vi "S4GUI_001.vi"() -> ()   [LabVIEW 2018] (continued)
                    n2026 = property on="Exptime ch3" class="DigNum (strict)"("Value"=w4669) -> ()  [unwired: 2 in, 2 out]
                  }
                }
                n2027 = call-dynamic "Read PREV_FT.vi"("error in (no error)"=w4601, "Interface in"=w4602) -> ("error out"=w4604:errorcluster, "PREV_FT"=w4603:bool, "Interface out"=w4605:refnum<class "Interface.lvclass">)  [unwired: 7 in]
                n2028 = call-dynamic "Get CCD_Config.vi"("error in (no error)"=w4604, "Interface in"=w4605) -> ("error out"=w4641:errorcluster, "output cluster"=w4640:T24, "Interface out"=w4644:refnum<class "Interface.lvclass">)  [unwired: 7 in]
                n2029 = Bundle By Name(cluster=w4640, "SHUTTER_MODE"=u8 1, "FRAME_TRANSFER"=w4603) -> (w4642:T24)
                n2030 = call-dynamic "Set CCD_Config.vi"("error in (no error)"=w4641, "input cluster"=w4642, "Interface in"=w4644) -> ("error out"=w4639:errorcluster, "Interface out"=w4645:refnum<class "Interface.lvclass">)  [unwired: 7 in]
                n2031 = Flatten To String(anything=w4642, error in (no error)=w4639) -> (data string=w4637:string, error out=w4638:errorcluster)  [unwired: 2 in, 1 out]
                n2032 = call "Write flatted cluster.vi"("error in (no error)"=w4638, "flatted cluster"=w4637, "Interface in"=w4645) -> ("error out"=w4647:errorcluster, "Interface out"=w4646:refnum<class "Interface.lvclass">)  [unwired: 7 in]
                n2033 = call-dynamic "Write Interface.vi"("error in (no error)"=w4647, "Interface.lvclass"=w4646, "Channel in"=w4633) -> ("error out"=w4652:errorcluster, "Channel out"=w4653:refnum<class "Channel.lvclass">)  [unwired: 7 in]
                n2034 = call "Write section_name.vi"("error in (no error)"=w4652, "section_name"="CCD_ACS3", "Channel in"=w4653) -> ("error out"=w4651:errorcluster, "Channel out"=w4656:refnum<class "Channel.lvclass">)  [unwired: 7 in]
                n2035 = call-dynamic "save config.vi"("error in (no error)"=w4651, "file config"="lastsaved.cfg", "Channel in"=w4656) -> ("error out"=w4610:errorcluster, "Channel out"=w4613:refnum<class "Channel.lvclass">)  [unwired: 7 in]
                n2036 = local read "Filter3"() -> (w4609:u8)
                n2037 = call-dynamic "Write Filter.vi"("error in (no error)"=w4610, "Filter"=w4609, "Channel in"=w4613) -> ("error out"=w4614:errorcluster, "Channel out"=w4627:refnum<class "Channel.lvclass">)  [unwired: 7 in]
                n2038 = call-dynamic "Read Interface.vi"("error in (no error)"=w4614, "Channel in"=w4627) -> ("error out"=w4617:errorcluster, "Interface.lvclass"=w4618:refnum<class "Interface.lvclass">, "Channel out"=w4628:refnum<class "Channel.lvclass">)  [unwired: 7 in]
                n2039 = call-dynamic "Write Suffix.vi"("error in (no error)"=w4617, "Suffix"=w4600, "Interface in"=w4618) -> ("error out"=w4626:errorcluster, "Interface out"=w4623:refnum<class "Interface.lvclass">)  [unwired: 7 in]
                n2040 = call-dynamic "Write ObsType.vi"("error in (no error)"=w4626, "ObsType"=w4599, "Interface in"=w4623) -> ("error out"=w4625:errorcluster, "Interface out"=w4622:refnum<class "Interface.lvclass">)  [unwired: 7 in]
                n2041 = call-dynamic "Write Object.vi"("error in (no error)"=w4625, "Object"=w4608, "Interface in"=w4622) -> ("error out"=w4624:errorcluster, "Interface out"=w4621:refnum<class "Interface.lvclass">)  [unwired: 7 in]
                n2042 = call-dynamic "Write Comments.vi"("error in (no error)"=w4624, "Comments"=w4607, "Interface in"=w4621) -> ("error out"=w4620:errorcluster, "Interface out"=w4619:refnum<class "Interface.lvclass">)  [unwired: 7 in]
                n2043 = call-dynamic "Write Observer.vi"("error in (no error)"=w4620, "Observer"=w4606, "Interface in"=w4619) -> ("error out"=w4615:errorcluster, "Interface out"=w4616:refnum<class "Interface.lvclass">)  [unwired: 7 in]
                n2044 = call-dynamic "Write Interface.vi"("error in (no error)"=w4615, "Interface.lvclass"=w4616, "Channel in"=w4628) -> ("error out"=w4611:errorcluster, "Channel out"=w4612:refnum<class "Channel.lvclass">)  [unwired: 7 in]
                n2045 = call-dynamic "Read State Machine.vi"("error in (no error)"=w4611, "Device in"=w4612) -> ("error out"=w4648:errorcluster, "State Machine.lvclass"=w4658:refnum<class "State Machine.lvclass">, "Device out"=w4657:refnum<class "Channel.lvclass">)  [unwired: 7 in]
                n2046 = call-dynamic "Write State.vi"("error in (no error)"=w4648, "State"=60, "State Machine in"=w4658) -> ("error out"=w4649:errorcluster, "State Machine out"=w4659:refnum<class "State Machine.lvclass">)  [unwired: 7 in]
                n2047 = call-dynamic "Write State Machine.vi"("error in (no error)"=w4649, "State Machine.lvclass"=w4659, "Device in"=w4657) -> ("error out"=w4661:errorcluster, "Device out"=w4660:refnum<class "Channel.lvclass">)  [unwired: 7 in]
                n2048 = call-dynamic "Write Channel.vi"("error in (no error)"=w4661, "Channel.lvclass"=w4660, "Acquisition in"=w4634) -> ("error out"=w4629:errorcluster, "Acquisition out"=w4630:refnum<class "Acquisition.lvclass">)  [unwired: 7 in]
              }
            }
          }
        }
        n2049 = call-dynamic "Write AcquisitionA.vi"("error in (no error)"=w3774, "Acquisition.lvclass"=w3775, "S4ACS_GUI in"=w3776) -> ("error out"=w3764:errorcluster, "S4ACS_GUI out"=w3768:refnum<class "S4GUI.lvclass">)  [unwired: 7 in]
        n2050 = call "Write AcquisitionB.vi"("error in (no error)"=w3769, "Acquisition.lvclass"=w3770, "S4ACS_GUI in"=w3768) -> ("error out"=w3763:errorcluster, "S4ACS_GUI out"=w3767:refnum<class "S4GUI.lvclass">)  [unwired: 7 in]
        n2051 = call-dynamic "Write AcquisitionC.vi"("error in (no error)"=w3758, "Acquisition.lvclass"=w3759, "S4ACS_GUI in"=w3767) -> ("error out"=w3762:errorcluster, "S4ACS_GUI out"=w3766:refnum<class "S4GUI.lvclass">)  [unwired: 7 in]
        n2052 = call-dynamic "Write AcquisitionD.vi"("error in (no error)"=w3756, "Acquisition.lvclass"=w3757, "S4ACS_GUI in"=w3766) -> ("error out"=w3761:errorcluster, "S4ACS_GUI out"=w3765:refnum<class "S4GUI.lvclass">)  [unwired: 7 in]
        n2053 = Merge Errors(w3764, w3763, w3762, w3761) -> (w3760:errorcluster)
        n2054 = call "Write cfg file.vi"("error in (no error)"=w3760, "cfg file"="lastsaved.cfg", "S4ACS_GUI in"=w3765) -> ("error out"=w3772:errorcluster, "S4ACS_GUI out"=w3771:refnum<class "S4GUI.lvclass">)  [unwired: 7 in]
      }
      event "set keywords": Value Change {
        # "SET Observer, suffix, comments e object da aba selecionada."
        n2055 = event-data() -> ()  [unwired: 1 in, 1 out]
        n2056 = local read "Tab Acq Type"() -> (w4846:T1)
        n2057 = local read "Observer"() -> (w4848:string)
        n2058 = case shown="\"ZERO\"" w4846 {
          tunnel: ["OBJECT" "FLAT" "FLAT" "DARK" "ZERO" "FOCUS"] -> w4852
          tunnel: [w5044 w5048 w5052 w5056 w5060 w5064] -> w4851
          tunnel: [w5043 w5047 w5051 w5055 w5059 w5063] -> w4850
          tunnel: [w5042 w5046 w5050 w5054 w5058 w5062] -> w4849
          frame "OBJECT", Default {
            n2059 = local read "Object_obj"() -> (w5044:string)
            n2060 = local read "OBJECT Comments"() -> (w5042:string)
            n2061 = local read "object suffix"() -> (w5043:string)
          }
          frame "DFLAT" {
            n2062 = local read "DFLAT Comments"() -> (w5046:string)
            n2063 = local read "Object_dflat"() -> (w5048:string)
            n2064 = local read "dflat suffix"() -> (w5047:string)
          }
          frame "SFLAT" {
            n2065 = local read "SFLAT Comments"() -> (w5050:string)
            n2066 = local read "Object_sflat"() -> (w5052:string)
            n2067 = local read "sflat suffix"() -> (w5051:string)
          }
          frame "DARK" {
            n2068 = local read "Object_dark"() -> (w5056:string)
            n2069 = local read "dark suffix"() -> (w5055:string)
            n2070 = local read "DARK Comments"() -> (w5054:string)
          }
          frame "ZERO" {
            n2071 = local read "ZERO Comments"() -> (w5058:string)
            n2072 = local read "Object_zero"() -> (w5060:string)
            n2073 = local read "zero suffix"() -> (w5059:string)
          }
          frame "FOCUS" {
            n2074 = local read "FOCUS Comments"() -> (w5062:string)
            n2075 = local read "Object_focus"() -> (w5064:string)
            n2076 = local read "focus suffix"() -> (w5063:string)
          }
        }
        n2077 = call-dynamic "Read AcquisitionC.vi"("error in (no error)"=w4832, "S4ACS_GUI in"=w4833) -> ("error out"=w4855:errorcluster, "Acquisition.lvclass"=w4856:refnum<class "Acquisition.lvclass">)  [unwired: 7 in, 1 out]
        n2078 = call-dynamic "Read AcquisitionA.vi"("error in (no error)"=w4832, "S4ACS_GUI in"=w4833) -> ("error out"=w4859:errorcluster, "Acquisition.lvclass"=w4860:refnum<class "Acquisition.lvclass">, "S4ACS_GUI out"=w4881:refnum<class "S4GUI.lvclass">)  [unwired: 7 in]
        n2079 = call "Read AcquisitionB.vi"("error in (no error)"=w4832, "S4ACS_GUI in"=w4833) -> ("error out"=w4857:errorcluster, "Acquisition.lvclass"=w4858:refnum<class "Acquisition.lvclass">)  [unwired: 7 in, 1 out]
        n2080 = call-dynamic "Read AcquisitionD.vi"("error in (no error)"=w4832, "S4ACS_GUI in"=w4833) -> ("error out"=w4853:errorcluster, "Acquisition.lvclass"=w4854:refnum<class "Acquisition.lvclass">)  [unwired: 7 in, 1 out]
        n2081 = call "Read connection.vi"("error in (no error)"=w4853, "Server in"=w4854) -> ("error out"=w4835:errorcluster, "connection"=w4834:bool, "Server out"=w4836:refnum<class "Acquisition.lvclass">)  [unwired: 7 in]
        n2082 = call "Read connection.vi"("error in (no error)"=w4855, "Server in"=w4856) -> ("error out"=w4838:errorcluster, "connection"=w4837:bool, "Server out"=w4839:refnum<class "Acquisition.lvclass">)  [unwired: 7 in]
        n2083 = call "Read connection.vi"("error in (no error)"=w4857, "Server in"=w4858) -> ("error out"=w4841:errorcluster, "connection"=w4840:bool, "Server out"=w4842:refnum<class "Acquisition.lvclass">)  [unwired: 7 in]
        n2084 = call "Read connection.vi"("error in (no error)"=w4859, "Server in"=w4860) -> ("error out"=w4844:errorcluster, "connection"=w4843:bool, "Server out"=w4845:refnum<class "Acquisition.lvclass">)  [unwired: 7 in]
        n2085 = To Lower Case(string=w4850) -> (all lower case string=w4847:string)
        n2086 = case shown="True" w4840 {
          tunnel: w4842 -> [w4963 w4992]
          tunnel: w4841 -> [w4962 w4991]
          tunnel: [w4963 w4990] -> w4875
          tunnel: [w4962 w4989] -> w4874
          tunnel: w4847 -> [_ w4970]
          tunnel: w4852 -> [_ w4969]
          tunnel: w4851 -> [_ w4968]
          tunnel: w4849 -> [_ w4967]
          tunnel: w4848 -> [_ w4966]
          frame False {
          }
          frame True {
            n2087 = call-dynamic "Read Channel.vi"("error in (no error)"=w4991, "Acquisition in"=w4992) -> ("error out"=w4964:errorcluster, "Channel.lvclass"=w4965:refnum<class "Channel.lvclass">, "Acquisition out"=w4993:refnum<class "Acquisition.lvclass">)  [unwired: 7 in]
            n2088 = local read "Filter2"() -> (w4971:u8)
            n2089 = call-dynamic "Write Filter.vi"("error in (no error)"=w4964, "Filter"=w4971, "Channel in"=w4965) -> ("error out"=w4988:errorcluster, "Channel out"=w4975:refnum<class "Channel.lvclass">)  [unwired: 7 in]
            n2090 = call-dynamic "Read Interface.vi"("error in (no error)"=w4988, "Channel in"=w4975) -> ("error out"=w4985:errorcluster, "Interface.lvclass"=w4984:refnum<class "Interface.lvclass">, "Channel out"=w4974:refnum<class "Channel.lvclass">)  [unwired: 7 in]
            n2091 = call-dynamic "Write Suffix.vi"("error in (no error)"=w4985, "Suffix"=w4970, "Interface in"=w4984) -> ("error out"=w4976:errorcluster, "Interface out"=w4979:refnum<class "Interface.lvclass">)  [unwired: 7 in]
            n2092 = call-dynamic "Write ObsType.vi"("error in (no error)"=w4976, "ObsType"=w4969, "Interface in"=w4979) -> ("error out"=w4977:errorcluster, "Interface out"=w4980:refnum<class "Interface.lvclass">)  [unwired: 7 in]
            n2093 = call-dynamic "Write Object.vi"("error in (no error)"=w4977, "Object"=w4968, "Interface in"=w4980) -> ("error out"=w4978:errorcluster, "Interface out"=w4981:refnum<class "Interface.lvclass">)  [unwired: 7 in]
            n2094 = call-dynamic "Write Comments.vi"("error in (no error)"=w4978, "Comments"=w4967, "Interface in"=w4981) -> ("error out"=w4982:errorcluster, "Interface out"=w4983:refnum<class "Interface.lvclass">)  [unwired: 7 in]
            n2095 = call-dynamic "Write Observer.vi"("error in (no error)"=w4982, "Observer"=w4966, "Interface in"=w4983) -> ("error out"=w4987:errorcluster, "Interface out"=w4986:refnum<class "Interface.lvclass">)  [unwired: 7 in]
            n2096 = call-dynamic "Write Interface.vi"("error in (no error)"=w4987, "Interface.lvclass"=w4986, "Channel in"=w4974) -> ("error out"=w4972:errorcluster, "Channel out"=w4973:refnum<class "Channel.lvclass">)  [unwired: 7 in]
            n2097 = call-dynamic "Read State Machine.vi"("error in (no error)"=w4972, "Device in"=w4973) -> ("error out"=w4994:errorcluster, "State Machine.lvclass"=w4998:refnum<class "State Machine.lvclass">, "Device out"=w4997:refnum<class "Channel.lvclass">)  [unwired: 7 in]
            n2098 = call-dynamic "Write State.vi"("error in (no error)"=w4994, "State"=12, "State Machine in"=w4998) -> ("error out"=w4995:errorcluster, "State Machine out"=w4999:refnum<class "State Machine.lvclass">)  [unwired: 7 in]
            n2099 = call-dynamic "Write State Machine.vi"("error in (no error)"=w4995, "State Machine.lvclass"=w4999, "Device in"=w4997) -> ("error out"=w5001:errorcluster, "Device out"=w5000:refnum<class "Channel.lvclass">)  [unwired: 7 in]
            n2100 = call-dynamic "Write Channel.vi"("error in (no error)"=w5001, "Channel.lvclass"=w5000, "Acquisition in"=w4993) -> ("error out"=w4989:errorcluster, "Acquisition out"=w4990:refnum<class "Acquisition.lvclass">)  [unwired: 7 in]
          }
        }
        n2101 = case shown="True" w4843 {
          tunnel: [w5002 w5040] -> w4879
          tunnel: [w5003 w5039] -> w4880
          tunnel: w4845 -> [w5003 w5030]
          tunnel: w4844 -> [w5002 w5029]
          tunnel: w4847 -> [_ w5010]
          tunnel: w4852 -> [_ w5009]
          tunnel: w4851 -> [_ w5008]
          tunnel: w4849 -> [_ w5007]
          tunnel: w4848 -> [_ w5006]
          frame False {
          }
          frame True {
            n2102 = call-dynamic "Read Channel.vi"("error in (no error)"=w5029, "Acquisition in"=w5030) -> ("error out"=w5004:errorcluster, "Channel.lvclass"=w5005:refnum<class "Channel.lvclass">, "Acquisition out"=w5041:refnum<class "Acquisition.lvclass">)  [unwired: 7 in]
            n2103 = local read "Filter1"() -> (w5013:u8)
            n2104 = call-dynamic "Write Filter.vi"("error in (no error)"=w5004, "Filter"=w5013, "Channel in"=w5005) -> ("error out"=w5028:errorcluster, "Channel out"=w5027:refnum<class "Channel.lvclass">)  [unwired: 7 in]
            n2105 = call-dynamic "Read Interface.vi"("error in (no error)"=w5028, "Channel in"=w5027) -> ("error out"=w5024:errorcluster, "Interface.lvclass"=w5023:refnum<class "Interface.lvclass">, "Channel out"=w5017:refnum<class "Channel.lvclass">)  [unwired: 7 in]
            n2106 = call-dynamic "Write Suffix.vi"("error in (no error)"=w5024, "Suffix"=w5010, "Interface in"=w5023) -> ("error out"=w5014:errorcluster, "Interface out"=w5018:refnum<class "Interface.lvclass">)  [unwired: 7 in]
            n2107 = call-dynamic "Write ObsType.vi"("error in (no error)"=w5014, "ObsType"=w5009, "Interface in"=w5018) -> ("error out"=w5015:errorcluster, "Interface out"=w5019:refnum<class "Interface.lvclass">)  [unwired: 7 in]
            n2108 = call-dynamic "Write Object.vi"("error in (no error)"=w5015, "Object"=w5008, "Interface in"=w5019) -> ("error out"=w5016:errorcluster, "Interface out"=w5020:refnum<class "Interface.lvclass">)  [unwired: 7 in]
            n2109 = call-dynamic "Write Comments.vi"("error in (no error)"=w5016, "Comments"=w5007, "Interface in"=w5020) -> ("error out"=w5021:errorcluster, "Interface out"=w5022:refnum<class "Interface.lvclass">)  [unwired: 7 in]
            n2110 = call-dynamic "Write Observer.vi"("error in (no error)"=w5021, "Observer"=w5006, "Interface in"=w5022) -> ("error out"=w5026:errorcluster, "Interface out"=w5025:refnum<class "Interface.lvclass">)  [unwired: 7 in]
            n2111 = call-dynamic "Write Interface.vi"("error in (no error)"=w5026, "Interface.lvclass"=w5025, "Channel in"=w5017) -> ("error out"=w5011:errorcluster, "Channel out"=w5012:refnum<class "Channel.lvclass">)  [unwired: 7 in]
            n2112 = call-dynamic "Read State Machine.vi"("error in (no error)"=w5011, "Device in"=w5012) -> ("error out"=w5038:errorcluster, "State Machine.lvclass"=w5034:refnum<class "State Machine.lvclass">, "Device out"=w5035:refnum<class "Channel.lvclass">)  [unwired: 7 in]
            n2113 = call-dynamic "Write State.vi"("error in (no error)"=w5038, "State"=12, "State Machine in"=w5034) -> ("error out"=w5037:errorcluster, "State Machine out"=w5033:refnum<class "State Machine.lvclass">)  [unwired: 7 in]
            n2114 = call-dynamic "Write State Machine.vi"("error in (no error)"=w5037, "State Machine.lvclass"=w5033, "Device in"=w5035) -> ("error out"=w5031:errorcluster, "Device out"=w5032:refnum<class "Channel.lvclass">)  [unwired: 7 in]
            n2115 = call-dynamic "Write Channel.vi"("error in (no error)"=w5031, "Channel.lvclass"=w5032, "Acquisition in"=w5041) -> ("error out"=w5040:errorcluster, "Acquisition out"=w5039:refnum<class "Acquisition.lvclass">)  [unwired: 7 in]
          }
        }
        n2116 = case shown="True" w4837 {
          tunnel: w4839 -> [w4923 w4952]
          tunnel: w4838 -> [w4922 w4951]
          tunnel: [w4923 w4950] -> w4864
          tunnel: [w4922 w4949] -> w4863
          tunnel: w4847 -> [_ w4930]
          tunnel: w4852 -> [_ w4929]
          tunnel: w4851 -> [_ w4928]
          tunnel: w4849 -> [_ w4927]
          tunnel: w4848 -> [_ w4926]
          frame False {
          }
          frame True {
            n2117 = call-dynamic "Read Channel.vi"("error in (no error)"=w4951, "Acquisition in"=w4952) -> ("error out"=w4924:errorcluster, "Channel.lvclass"=w4925:refnum<class "Channel.lvclass">, "Acquisition out"=w4953:refnum<class "Acquisition.lvclass">)  [unwired: 7 in]
            n2118 = local read "Filter3"() -> (w4931:u8)
            n2119 = call-dynamic "Write Filter.vi"("error in (no error)"=w4924, "Filter"=w4931, "Channel in"=w4925) -> ("error out"=w4934:errorcluster, "Channel out"=w4947:refnum<class "Channel.lvclass">)  [unwired: 7 in]
            n2120 = call-dynamic "Read Interface.vi"("error in (no error)"=w4934, "Channel in"=w4947) -> ("error out"=w4937:errorcluster, "Interface.lvclass"=w4938:refnum<class "Interface.lvclass">, "Channel out"=w4948:refnum<class "Channel.lvclass">)  [unwired: 7 in]
            n2121 = call-dynamic "Write Suffix.vi"("error in (no error)"=w4937, "Suffix"=w4930, "Interface in"=w4938) -> ("error out"=w4946:errorcluster, "Interface out"=w4943:refnum<class "Interface.lvclass">)  [unwired: 7 in]
            n2122 = call-dynamic "Write ObsType.vi"("error in (no error)"=w4946, "ObsType"=w4929, "Interface in"=w4943) -> ("error out"=w4945:errorcluster, "Interface out"=w4942:refnum<class "Interface.lvclass">)  [unwired: 7 in]
            n2123 = call-dynamic "Write Object.vi"("error in (no error)"=w4945, "Object"=w4928, "Interface in"=w4942) -> ("error out"=w4944:errorcluster, "Interface out"=w4941:refnum<class "Interface.lvclass">)  [unwired: 7 in]
            n2124 = call-dynamic "Write Comments.vi"("error in (no error)"=w4944, "Comments"=w4927, "Interface in"=w4941) -> ("error out"=w4940:errorcluster, "Interface out"=w4939:refnum<class "Interface.lvclass">)  [unwired: 7 in]
            n2125 = call-dynamic "Write Observer.vi"("error in (no error)"=w4940, "Observer"=w4926, "Interface in"=w4939) -> ("error out"=w4935:errorcluster, "Interface out"=w4936:refnum<class "Interface.lvclass">)  [unwired: 7 in]
            n2126 = call-dynamic "Write Interface.vi"("error in (no error)"=w4935, "Interface.lvclass"=w4936, "Channel in"=w4948) -> ("error out"=w4932:errorcluster, "Channel out"=w4933:refnum<class "Channel.lvclass">)  [unwired: 7 in]
            n2127 = call-dynamic "Read State Machine.vi"("error in (no error)"=w4932, "Device in"=w4933) -> ("error out"=w4954:errorcluster, "State Machine.lvclass"=w4958:refnum<class "State Machine.lvclass">, "Device out"=w4957:refnum<class "Channel.lvclass">)  [unwired: 7 in]
            n2128 = call-dynamic "Write State.vi"("error in (no error)"=w4954, "State"=12, "State Machine in"=w4958) -> ("error out"=w4955:errorcluster, "State Machine out"=w4959:refnum<class "State Machine.lvclass">)  [unwired: 7 in]
            n2129 = call-dynamic "Write State Machine.vi"("error in (no error)"=w4955, "State Machine.lvclass"=w4959, "Device in"=w4957) -> ("error out"=w4961:errorcluster, "Device out"=w4960:refnum<class "Channel.lvclass">)  [unwired: 7 in]
            n2130 = call-dynamic "Write Channel.vi"("error in (no error)"=w4961, "Channel.lvclass"=w4960, "Acquisition in"=w4953) -> ("error out"=w4949:errorcluster, "Acquisition out"=w4950:refnum<class "Acquisition.lvclass">)  [unwired: 7 in]
          }
        }
        n2131 = case shown="True" w4834 {
          tunnel: w4836 -> [w4883 w4912]
          tunnel: w4835 -> [w4882 w4911]
          tunnel: [w4883 w4910] -> w4862
          tunnel: [w4882 w4909] -> w4861
          tunnel: w4847 -> [_ w4890]
          tunnel: w4852 -> [_ w4889]
          tunnel: w4851 -> [_ w4888]
          tunnel: w4849 -> [_ w4887]
          tunnel: w4848 -> [_ w4886]
          frame False {
          }
          frame True {
            n2132 = call-dynamic "Read Channel.vi"("error in (no error)"=w4911, "Acquisition in"=w4912) -> ("error out"=w4884:errorcluster, "Channel.lvclass"=w4885:refnum<class "Channel.lvclass">, "Acquisition out"=w4921:refnum<class "Acquisition.lvclass">)  [unwired: 7 in]
            n2133 = local read "Filter4"() -> (w4891:u8)
            n2134 = call-dynamic "Write Filter.vi"("error in (no error)"=w4884, "Filter"=w4891, "Channel in"=w4885) -> ("error out"=w4908:errorcluster, "Channel out"=w4895:refnum<class "Channel.lvclass">)  [unwired: 7 in]
            n2135 = call-dynamic "Read Interface.vi"("error in (no error)"=w4908, "Channel in"=w4895) -> ("error out"=w4905:errorcluster, "Interface.lvclass"=w4904:refnum<class "Interface.lvclass">, "Channel out"=w4894:refnum<class "Channel.lvclass">)  [unwired: 7 in]
            n2136 = call-dynamic "Write Suffix.vi"("error in (no error)"=w4905, "Suffix"=w4890, "Interface in"=w4904) -> ("error out"=w4896:errorcluster, "Interface out"=w4899:refnum<class "Interface.lvclass">)  [unwired: 7 in]
            n2137 = call-dynamic "Write ObsType.vi"("error in (no error)"=w4896, "ObsType"=w4889, "Interface in"=w4899) -> ("error out"=w4897:errorcluster, "Interface out"=w4900:refnum<class "Interface.lvclass">)  [unwired: 7 in]
            n2138 = call-dynamic "Write Object.vi"("error in (no error)"=w4897, "Object"=w4888, "Interface in"=w4900) -> ("error out"=w4898:errorcluster, "Interface out"=w4901:refnum<class "Interface.lvclass">)  [unwired: 7 in]
            n2139 = call-dynamic "Write Comments.vi"("error in (no error)"=w4898, "Comments"=w4887, "Interface in"=w4901) -> ("error out"=w4902:errorcluster, "Interface out"=w4903:refnum<class "Interface.lvclass">)  [unwired: 7 in]
            n2140 = call-dynamic "Write Observer.vi"("error in (no error)"=w4902, "Observer"=w4886, "Interface in"=w4903) -> ("error out"=w4907:errorcluster, "Interface out"=w4906:refnum<class "Interface.lvclass">)  [unwired: 7 in]
            n2141 = call-dynamic "Write Interface.vi"("error in (no error)"=w4907, "Interface.lvclass"=w4906, "Channel in"=w4894) -> ("error out"=w4892:errorcluster, "Channel out"=w4893:refnum<class "Channel.lvclass">)  [unwired: 7 in]
            n2142 = call-dynamic "Read State Machine.vi"("error in (no error)"=w4892, "Device in"=w4893) -> ("error out"=w4920:errorcluster, "State Machine.lvclass"=w4916:refnum<class "State Machine.lvclass">, "Device out"=w4917:refnum<class "Channel.lvclass">)  [unwired: 7 in]
            n2143 = call-dynamic "Write State.vi"("error in (no error)"=w4920, "State"=12, "State Machine in"=w4916) -> ("error out"=w4919:errorcluster, "State Machine out"=w4915:refnum<class "State Machine.lvclass">)  [unwired: 7 in]
            n2144 = call-dynamic "Write State Machine.vi"("error in (no error)"=w4919, "State Machine.lvclass"=w4915, "Device in"=w4917) -> ("error out"=w4913:errorcluster, "Device out"=w4914:refnum<class "Channel.lvclass">)  [unwired: 7 in]
            n2145 = call-dynamic "Write Channel.vi"("error in (no error)"=w4913, "Channel.lvclass"=w4914, "Acquisition in"=w4921) -> ("error out"=w4909:errorcluster, "Acquisition out"=w4910:refnum<class "Acquisition.lvclass">)  [unwired: 7 in]
          }
        }
        n2146 = call-dynamic "Write AcquisitionA.vi"("error in (no error)"=w4879, "Acquisition.lvclass"=w4880, "S4ACS_GUI in"=w4881) -> ("error out"=w4869:errorcluster, "S4ACS_GUI out"=w4873:refnum<class "S4GUI.lvclass">)  [unwired: 7 in]
        n2147 = call "Write AcquisitionB.vi"("error in (no error)"=w4874, "Acquisition.lvclass"=w4875, "S4ACS_GUI in"=w4873) -> ("error out"=w4868:errorcluster, "S4ACS_GUI out"=w4872:refnum<class "S4GUI.lvclass">)  [unwired: 7 in]
        n2148 = call-dynamic "Write AcquisitionC.vi"("error in (no error)"=w4863, "Acquisition.lvclass"=w4864, "S4ACS_GUI in"=w4872) -> ("error out"=w4867:errorcluster, "S4ACS_GUI out"=w4871:refnum<class "S4GUI.lvclass">)  [unwired: 7 in]
        n2149 = call-dynamic "Write AcquisitionD.vi"("error in (no error)"=w4861, "Acquisition.lvclass"=w4862, "S4ACS_GUI in"=w4871) -> ("error out"=w4866:errorcluster, "S4ACS_GUI out"=w4870:refnum<class "S4GUI.lvclass">)  [unwired: 7 in]
        n2150 = Merge Errors(w4869, w4868, w4867, w4866) -> (w4865:errorcluster)
        n2151 = call "Write cfg file.vi"("error in (no error)"=w4865, "cfg file"="lastsaved.cfg", "S4ACS_GUI in"=w4870) -> ("error out"=w4877:errorcluster, "S4ACS_GUI out"=w4876:refnum<class "S4GUI.lvclass">)  [unwired: 7 in]
      }
      event "Object_sflat", "Object_dark", "Object_zero", "Object_dflat", "Object_focus", "Object_obj": Value Change {
        n2152 = event-data() -> ("NewVal"=w5066:string)  [unwired: 1 in, 5 out]
        n2153 = stacked-sequence {
          seq-local: [w5102 _ _ _] -> [_ w5160 _ _]
          seq-local: [w5101 _ _ _] -> [_ w5159 _ _]
          seq-local: [_ w5158 _ _] -> [_ _ w5203 _]
          seq-local: [_ w5157 _ _] -> [_ _ w5202 _]
          seq-local: [_ _ w5201 _] -> [_ _ _ w5246]
          seq-local: [_ _ w5200 _] -> [_ _ _ w5245]
          tunnel: w5073 -> [w5114 _ _ _]
          tunnel: w5074 -> [w5113 _ _ _]
          tunnel: [_ _ _ w5244] -> w5068
          tunnel: [_ _ _ w5243] -> w5067
          tunnel: w5072 -> [w5100 w5156 w5199 w5242]
          tunnel: w5071 -> [w5099 w5155 w5185 w5228]
          tunnel: w5069 -> [w5098 w5141 w5184 w5227]
          tunnel: w5066 -> [w5097 w5140 w5183 w5226]
          tunnel: w5070 -> [w5096 w5139 w5182 w5225]
          frame #0 {
            # "observer"
            # "comment"
            # "object"
            # "suffix"
            # "obsType"
            n2154 = call-dynamic "Read AcquisitionA.vi"("error in (no error)"=w5114, "S4ACS_GUI in"=w5113) -> ("error out"=w5112:errorcluster, "Acquisition.lvclass"=w5111:refnum<class "Acquisition.lvclass">, "S4ACS_GUI out"=w5106:refnum<class "S4GUI.lvclass">)  [unwired: 7 in]
            n2155 = call-dynamic "Read Channel.vi"("error in (no error)"=w5112, "Acquisition in"=w5111) -> ("error out"=w5076:errorcluster, "Channel.lvclass"=w5079:refnum<class "Channel.lvclass">, "Acquisition out"=w5105:refnum<class "Acquisition.lvclass">)  [unwired: 7 in]
            n2156 = local read "Filter1"() -> (w5077:u8)
            n2157 = call-dynamic "Write Filter.vi"("error in (no error)"=w5076, "Filter"=w5077, "Channel in"=w5079) -> ("error out"=w5075:errorcluster, "Channel out"=w5078:refnum<class "Channel.lvclass">)  [unwired: 7 in]
            n2158 = call-dynamic "Read Interface.vi"("error in (no error)"=w5075, "Channel in"=w5078) -> ("error out"=w5092:errorcluster, "Interface.lvclass"=w5093:refnum<class "Interface.lvclass">, "Channel out"=w5110:refnum<class "Channel.lvclass">)  [unwired: 7 in]
            n2159 = call-dynamic "Write Suffix.vi"("error in (no error)"=w5092, "Suffix"=w5100, "Interface in"=w5093) -> ("error out"=w5117:errorcluster, "Interface out"=w5109:refnum<class "Interface.lvclass">)  [unwired: 7 in]
            n2160 = call-dynamic "Write ObsType.vi"("error in (no error)"=w5117, "ObsType"=w5098, "Interface in"=w5109) -> ("error out"=w5116:errorcluster, "Interface out"=w5108:refnum<class "Interface.lvclass">)  [unwired: 7 in]
            n2161 = call-dynamic "Write Object.vi"("error in (no error)"=w5116, "Object"=w5097, "Interface in"=w5108) -> ("error out"=w5115:errorcluster, "Interface out"=w5107:refnum<class "Interface.lvclass">)  [unwired: 7 in]
            n2162 = call-dynamic "Write Comments.vi"("error in (no error)"=w5115, "Comments"=w5099, "Interface in"=w5107) -> ("error out"=w5095:errorcluster, "Interface out"=w5094:refnum<class "Interface.lvclass">)  [unwired: 7 in]
            n2163 = call-dynamic "Write Observer.vi"("error in (no error)"=w5095, "Observer"=w5096, "Interface in"=w5094) -> ("error out"=w5090:errorcluster, "Interface out"=w5091:refnum<class "Interface.lvclass">)  [unwired: 7 in]
            n2164 = call-dynamic "Write Interface.vi"("error in (no error)"=w5090, "Interface.lvclass"=w5091, "Channel in"=w5110) -> ("error out"=w5086:errorcluster, "Channel out"=w5089:refnum<class "Channel.lvclass">)  [unwired: 7 in]
            n2165 = call-dynamic "Read State Machine.vi"("error in (no error)"=w5086, "Device in"=w5089) -> ("error out"=w5085:errorcluster, "State Machine.lvclass"=w5083:refnum<class "State Machine.lvclass">, "Device out"=w5088:refnum<class "Channel.lvclass">)  [unwired: 7 in]
            n2166 = call "Next State.vi"("error in (no error)"=w5085, "New_State"=12, "State Machine in"=w5083) -> ("error out"=w5084:errorcluster, "State Machine out"=w5082:refnum<class "State Machine.lvclass">)  [unwired: 7 in]
            n2167 = call-dynamic "Write State Machine.vi"("error in (no error)"=w5084, "State Machine.lvclass"=w5082, "Device in"=w5088) -> ("error out"=w5081:errorcluster, "Device out"=w5087:refnum<class "Channel.lvclass">)  [unwired: 7 in]
            n2168 = call-dynamic "Write Channel.vi"("error in (no error)"=w5081, "Channel.lvclass"=w5087, "Acquisition in"=w5105) -> ("error out"=w5103:errorcluster, "Acquisition out"=w5104:refnum<class "Acquisition.lvclass">)  [unwired: 7 in]
            n2169 = call-dynamic "Write AcquisitionA.vi"("error in (no error)"=w5103, "Acquisition.lvclass"=w5104, "S4ACS_GUI in"=w5106) -> ("error out"=w5101:errorcluster, "S4ACS_GUI out"=w5102:refnum<class "S4GUI.lvclass">)  [unwired: 7 in]
          }
          frame #1 {
            # "object"
            # "suffix"
            # "obsType"
            n2170 = call "Read AcquisitionB.vi"("error in (no error)"=w5159, "S4ACS_GUI in"=w5160) -> ("error out"=w5145:errorcluster, "Acquisition.lvclass"=w5146:refnum<class "Acquisition.lvclass">, "S4ACS_GUI out"=w5151:refnum<class "S4GUI.lvclass">)  [unwired: 7 in]
            n2171 = call-dynamic "Read Channel.vi"("error in (no error)"=w5145, "Acquisition in"=w5146) -> ("error out"=w5119:errorcluster, "Channel.lvclass"=w5121:refnum<class "Channel.lvclass">, "Acquisition out"=w5152:refnum<class "Acquisition.lvclass">)  [unwired: 7 in]
            n2172 = local read "Filter2"() -> (w5122:u8)
            n2173 = call-dynamic "Write Filter.vi"("error in (no error)"=w5119, "Filter"=w5122, "Channel in"=w5121) -> ("error out"=w5118:errorcluster, "Channel out"=w5120:refnum<class "Channel.lvclass">)  [unwired: 7 in]
            n2174 = call-dynamic "Read Interface.vi"("error in (no error)"=w5118, "Channel in"=w5120) -> ("error out"=w5133:errorcluster, "Interface.lvclass"=w5134:refnum<class "Interface.lvclass">, "Channel out"=w5147:refnum<class "Channel.lvclass">)  [unwired: 7 in]
            n2175 = call-dynamic "Write Suffix.vi"("error in (no error)"=w5133, "Suffix"=w5156, "Interface in"=w5134) -> ("error out"=w5142:errorcluster, "Interface out"=w5148:refnum<class "Interface.lvclass">)  [unwired: 7 in]
            n2176 = call-dynamic "Write ObsType.vi"("error in (no error)"=w5142, "ObsType"=w5141, "Interface in"=w5148) -> ("error out"=w5143:errorcluster, "Interface out"=w5149:refnum<class "Interface.lvclass">)  [unwired: 7 in]
            n2177 = call-dynamic "Write Object.vi"("error in (no error)"=w5143, "Object"=w5140, "Interface in"=w5149) -> ("error out"=w5144:errorcluster, "Interface out"=w5150:refnum<class "Interface.lvclass">)  [unwired: 7 in]
            n2178 = call-dynamic "Write Comments.vi"("error in (no error)"=w5144, "Comments"=w5155, "Interface in"=w5150) -> ("error out"=w5136:errorcluster, "Interface out"=w5135:refnum<class "Interface.lvclass">)  [unwired: 7 in]
            n2179 = call-dynamic "Write Observer.vi"("error in (no error)"=w5136, "Observer"=w5139, "Interface in"=w5135) -> ("error out"=w5137:errorcluster, "Interface out"=w5138:refnum<class "Interface.lvclass">)  [unwired: 7 in]
            n2180 = call-dynamic "Write Interface.vi"("error in (no error)"=w5137, "Interface.lvclass"=w5138, "Channel in"=w5147) -> ("error out"=w5126:errorcluster, "Channel out"=w5127:refnum<class "Channel.lvclass">)  [unwired: 7 in]
            n2181 = call-dynamic "Read State Machine.vi"("error in (no error)"=w5126, "Device in"=w5127) -> ("error out"=w5132:errorcluster, "State Machine.lvclass"=w5130:refnum<class "State Machine.lvclass">, "Device out"=w5125:refnum<class "Channel.lvclass">)  [unwired: 7 in]
            n2182 = call "Next State.vi"("error in (no error)"=w5132, "New_State"=12, "State Machine in"=w5130) -> ("error out"=w5131:errorcluster, "State Machine out"=w5129:refnum<class "State Machine.lvclass">)  [unwired: 7 in]
            n2183 = call-dynamic "Write State Machine.vi"("error in (no error)"=w5131, "State Machine.lvclass"=w5129, "Device in"=w5125) -> ("error out"=w5123:errorcluster, "Device out"=w5124:refnum<class "Channel.lvclass">)  [unwired: 7 in]
            n2184 = call-dynamic "Write Channel.vi"("error in (no error)"=w5123, "Channel.lvclass"=w5124, "Acquisition in"=w5152) -> ("error out"=w5154:errorcluster, "Acquisition out"=w5153:refnum<class "Acquisition.lvclass">)  [unwired: 7 in]
            n2185 = call "Write AcquisitionB.vi"("error in (no error)"=w5154, "Acquisition.lvclass"=w5153, "S4ACS_GUI in"=w5151) -> ("error out"=w5157:errorcluster, "S4ACS_GUI out"=w5158:refnum<class "S4GUI.lvclass">)  [unwired: 7 in]
          }
          frame #2 {
            # "object"
            # "suffix"
            # "obsType"
            n2186 = call-dynamic "Read AcquisitionC.vi"("error in (no error)"=w5202, "S4ACS_GUI in"=w5203) -> ("error out"=w5195:errorcluster, "Acquisition.lvclass"=w5194:refnum<class "Acquisition.lvclass">, "S4ACS_GUI out"=w5189:refnum<class "S4GUI.lvclass">)  [unwired: 7 in]
            n2187 = call-dynamic "Read Channel.vi"("error in (no error)"=w5195, "Acquisition in"=w5194) -> ("error out"=w5162:errorcluster, "Channel.lvclass"=w5164:refnum<class "Channel.lvclass">, "Acquisition out"=w5188:refnum<class "Acquisition.lvclass">)  [unwired: 7 in]
            n2188 = local read "Filter3"() -> (w5165:u8)
            n2189 = call-dynamic "Write Filter.vi"("error in (no error)"=w5162, "Filter"=w5165, "Channel in"=w5164) -> ("error out"=w5161:errorcluster, "Channel out"=w5163:refnum<class "Channel.lvclass">)  [unwired: 7 in]
            n2190 = call-dynamic "Read Interface.vi"("error in (no error)"=w5161, "Channel in"=w5163) -> ("error out"=w5180:errorcluster, "Interface.lvclass"=w5181:refnum<class "Interface.lvclass">, "Channel out"=w5193:refnum<class "Channel.lvclass">)  [unwired: 7 in]
            n2191 = call-dynamic "Write Suffix.vi"("error in (no error)"=w5180, "Suffix"=w5199, "Interface in"=w5181) -> ("error out"=w5198:errorcluster, "Interface out"=w5192:refnum<class "Interface.lvclass">)  [unwired: 7 in]
            n2192 = call-dynamic "Write ObsType.vi"("error in (no error)"=w5198, "ObsType"=w5184, "Interface in"=w5192) -> ("error out"=w5197:errorcluster, "Interface out"=w5191:refnum<class "Interface.lvclass">)  [unwired: 7 in]
            n2193 = call-dynamic "Write Object.vi"("error in (no error)"=w5197, "Object"=w5183, "Interface in"=w5191) -> ("error out"=w5196:errorcluster, "Interface out"=w5190:refnum<class "Interface.lvclass">)  [unwired: 7 in]
            n2194 = call-dynamic "Write Comments.vi"("error in (no error)"=w5196, "Comments"=w5185, "Interface in"=w5190) -> ("error out"=w5177:errorcluster, "Interface out"=w5176:refnum<class "Interface.lvclass">)  [unwired: 7 in]
            n2195 = call-dynamic "Write Observer.vi"("error in (no error)"=w5177, "Observer"=w5182, "Interface in"=w5176) -> ("error out"=w5178:errorcluster, "Interface out"=w5179:refnum<class "Interface.lvclass">)  [unwired: 7 in]
            n2196 = call-dynamic "Write Interface.vi"("error in (no error)"=w5178, "Interface.lvclass"=w5179, "Channel in"=w5193) -> ("error out"=w5171:errorcluster, "Channel out"=w5172:refnum<class "Channel.lvclass">)  [unwired: 7 in]
            n2197 = call-dynamic "Read State Machine.vi"("error in (no error)"=w5171, "Device in"=w5172) -> ("error out"=w5175:errorcluster, "State Machine.lvclass"=w5168:refnum<class "State Machine.lvclass">, "Device out"=w5170:refnum<class "Channel.lvclass">)  [unwired: 7 in]
            n2198 = call "Next State.vi"("error in (no error)"=w5175, "New_State"=12, "State Machine in"=w5168) -> ("error out"=w5174:errorcluster, "State Machine out"=w5167:refnum<class "State Machine.lvclass">)  [unwired: 7 in]
            n2199 = call-dynamic "Write State Machine.vi"("error in (no error)"=w5174, "State Machine.lvclass"=w5167, "Device in"=w5170) -> ("error out"=w5166:errorcluster, "Device out"=w5169:refnum<class "Channel.lvclass">)  [unwired: 7 in]
            n2200 = call-dynamic "Write Channel.vi"("error in (no error)"=w5166, "Channel.lvclass"=w5169, "Acquisition in"=w5188) -> ("error out"=w5186:errorcluster, "Acquisition out"=w5187:refnum<class "Acquisition.lvclass">)  [unwired: 7 in]
            n2201 = call-dynamic "Write AcquisitionC.vi"("error in (no error)"=w5186, "Acquisition.lvclass"=w5187, "S4ACS_GUI in"=w5189) -> ("error out"=w5200:errorcluster, "S4ACS_GUI out"=w5201:refnum<class "S4GUI.lvclass">)  [unwired: 7 in]
          }
          frame #3 {
            # "object"
            # "suffix"
            # "obsType"
            n2202 = call-dynamic "Read AcquisitionD.vi"("error in (no error)"=w5245, "S4ACS_GUI in"=w5246) -> ("error out"=w5238:errorcluster, "Acquisition.lvclass"=w5237:refnum<class "Acquisition.lvclass">, "S4ACS_GUI out"=w5232:refnum<class "S4GUI.lvclass">)  [unwired: 7 in]
            n2203 = call-dynamic "Read Channel.vi"("error in (no error)"=w5238, "Acquisition in"=w5237) -> ("error out"=w5205:errorcluster, "Channel.lvclass"=w5207:refnum<class "Channel.lvclass">, "Acquisition out"=w5231:refnum<class "Acquisition.lvclass">)  [unwired: 7 in]
            n2204 = local read "Filter4"() -> (w5208:u8)
            n2205 = call-dynamic "Write Filter.vi"("error in (no error)"=w5205, "Filter"=w5208, "Channel in"=w5207) -> ("error out"=w5204:errorcluster, "Channel out"=w5206:refnum<class "Channel.lvclass">)  [unwired: 7 in]
            n2206 = call-dynamic "Read Interface.vi"("error in (no error)"=w5204, "Channel in"=w5206) -> ("error out"=w5223:errorcluster, "Interface.lvclass"=w5224:refnum<class "Interface.lvclass">, "Channel out"=w5236:refnum<class "Channel.lvclass">)  [unwired: 7 in]
            n2207 = call-dynamic "Write Suffix.vi"("error in (no error)"=w5223, "Suffix"=w5242, "Interface in"=w5224) -> ("error out"=w5241:errorcluster, "Interface out"=w5235:refnum<class "Interface.lvclass">)  [unwired: 7 in]
            n2208 = call-dynamic "Write ObsType.vi"("error in (no error)"=w5241, "ObsType"=w5227, "Interface in"=w5235) -> ("error out"=w5240:errorcluster, "Interface out"=w5234:refnum<class "Interface.lvclass">)  [unwired: 7 in]
            n2209 = call-dynamic "Write Object.vi"("error in (no error)"=w5240, "Object"=w5226, "Interface in"=w5234) -> ("error out"=w5239:errorcluster, "Interface out"=w5233:refnum<class "Interface.lvclass">)  [unwired: 7 in]
            n2210 = call-dynamic "Write Comments.vi"("error in (no error)"=w5239, "Comments"=w5228, "Interface in"=w5233) -> ("error out"=w5222:errorcluster, "Interface out"=w5221:refnum<class "Interface.lvclass">)  [unwired: 7 in]
            n2211 = call-dynamic "Write Observer.vi"("error in (no error)"=w5222, "Observer"=w5225, "Interface in"=w5221) -> ("error out"=w5217:errorcluster, "Interface out"=w5216:refnum<class "Interface.lvclass">)  [unwired: 7 in]
            n2212 = call-dynamic "Write Interface.vi"("error in (no error)"=w5217, "Interface.lvclass"=w5216, "Channel in"=w5236) -> ("error out"=w5212:errorcluster, "Channel out"=w5215:refnum<class "Channel.lvclass">)  [unwired: 7 in]
            n2213 = call-dynamic "Read State Machine.vi"("error in (no error)"=w5212, "Device in"=w5215) -> ("error out"=w5220:errorcluster, "State Machine.lvclass"=w5210:refnum<class "State Machine.lvclass">, "Device out"=w5214:refnum<class "Channel.lvclass">)  [unwired: 7 in]
            n2214 = call "Next State.vi"("error in (no error)"=w5220, "New_State"=12, "State Machine in"=w5210) -> ("error out"=w5219:errorcluster, "State Machine out"=w5209:refnum<class "State Machine.lvclass">)  [unwired: 7 in]
            n2215 = call-dynamic "Write State Machine.vi"("error in (no error)"=w5219, "State Machine.lvclass"=w5209, "Device in"=w5214) -> ("error out"=w5211:errorcluster, "Device out"=w5213:refnum<class "Channel.lvclass">)  [unwired: 7 in]
            n2216 = call-dynamic "Write Channel.vi"("error in (no error)"=w5211, "Channel.lvclass"=w5213, "Acquisition in"=w5231) -> ("error out"=w5229:errorcluster, "Acquisition out"=w5230:refnum<class "Acquisition.lvclass">)  [unwired: 7 in]
            n2217 = call-dynamic "Write AcquisitionD.vi"("error in (no error)"=w5229, "Acquisition.lvclass"=w5230, "S4ACS_GUI in"=w5232) -> ("error out"=w5243:errorcluster, "S4ACS_GUI out"=w5244:refnum<class "S4GUI.lvclass">)  [unwired: 7 in]
          }
        }
      }
      event "DFLAT Comments", "SFLAT Comments", "DARK Comments", "ZERO Comments", "FOCUS Comments", "OBJECT Comments": Value Change {
        n2218 = event-data() -> ("NewVal"=w5247:string)  [unwired: 1 in, 5 out]
        n2219 = stacked-sequence {
          seq-local: [w5283 _ _ _] -> [_ w5341 _ _]
          seq-local: [w5282 _ _ _] -> [_ w5340 _ _]
          seq-local: [_ w5339 _ _] -> [_ _ w5384 _]
          seq-local: [_ w5338 _ _] -> [_ _ w5383 _]
          seq-local: [_ _ w5382 _] -> [_ _ _ w5427]
          seq-local: [_ _ w5381 _] -> [_ _ _ w5426]
          tunnel: w5254 -> [w5295 _ _ _]
          tunnel: w5255 -> [w5294 _ _ _]
          tunnel: [_ _ _ w5425] -> w5249
          tunnel: [_ _ _ w5424] -> w5248
          tunnel: w5252 -> [w5281 w5337 w5380 w5423]
          tunnel: w5247 -> [w5280 w5336 w5366 w5409]
          tunnel: w5250 -> [w5279 w5322 w5365 w5408]
          tunnel: w5253 -> [w5278 w5321 w5364 w5407]
          tunnel: w5251 -> [w5277 w5320 w5363 w5406]
          frame #0 {
            # "observer"
            # "comment"
            # "object"
            # "suffix"
            # "obsType"
            n2220 = call-dynamic "Read AcquisitionA.vi"("error in (no error)"=w5295, "S4ACS_GUI in"=w5294) -> ("error out"=w5293:errorcluster, "Acquisition.lvclass"=w5292:refnum<class "Acquisition.lvclass">, "S4ACS_GUI out"=w5287:refnum<class "S4GUI.lvclass">)  [unwired: 7 in]
            n2221 = call-dynamic "Read Channel.vi"("error in (no error)"=w5293, "Acquisition in"=w5292) -> ("error out"=w5257:errorcluster, "Channel.lvclass"=w5260:refnum<class "Channel.lvclass">, "Acquisition out"=w5286:refnum<class "Acquisition.lvclass">)  [unwired: 7 in]
            n2222 = local read "Filter1"() -> (w5258:u8)
            n2223 = call-dynamic "Write Filter.vi"("error in (no error)"=w5257, "Filter"=w5258, "Channel in"=w5260) -> ("error out"=w5256:errorcluster, "Channel out"=w5259:refnum<class "Channel.lvclass">)  [unwired: 7 in]
            n2224 = call-dynamic "Read Interface.vi"("error in (no error)"=w5256, "Channel in"=w5259) -> ("error out"=w5273:errorcluster, "Interface.lvclass"=w5274:refnum<class "Interface.lvclass">, "Channel out"=w5291:refnum<class "Channel.lvclass">)  [unwired: 7 in]
            n2225 = call-dynamic "Write Suffix.vi"("error in (no error)"=w5273, "Suffix"=w5281, "Interface in"=w5274) -> ("error out"=w5298:errorcluster, "Interface out"=w5290:refnum<class "Interface.lvclass">)  [unwired: 7 in]
            n2226 = call-dynamic "Write ObsType.vi"("error in (no error)"=w5298, "ObsType"=w5279, "Interface in"=w5290) -> ("error out"=w5297:errorcluster, "Interface out"=w5289:refnum<class "Interface.lvclass">)  [unwired: 7 in]
            n2227 = call-dynamic "Write Object.vi"("error in (no error)"=w5297, "Object"=w5278, "Interface in"=w5289) -> ("error out"=w5296:errorcluster, "Interface out"=w5288:refnum<class "Interface.lvclass">)  [unwired: 7 in]
            n2228 = call-dynamic "Write Comments.vi"("error in (no error)"=w5296, "Comments"=w5280, "Interface in"=w5288) -> ("error out"=w5276:errorcluster, "Interface out"=w5275:refnum<class "Interface.lvclass">)  [unwired: 7 in]
            n2229 = call-dynamic "Write Observer.vi"("error in (no error)"=w5276, "Observer"=w5277, "Interface in"=w5275) -> ("error out"=w5271:errorcluster, "Interface out"=w5272:refnum<class "Interface.lvclass">)  [unwired: 7 in]
            n2230 = call-dynamic "Write Interface.vi"("error in (no error)"=w5271, "Interface.lvclass"=w5272, "Channel in"=w5291) -> ("error out"=w5267:errorcluster, "Channel out"=w5270:refnum<class "Channel.lvclass">)  [unwired: 7 in]
            n2231 = call-dynamic "Read State Machine.vi"("error in (no error)"=w5267, "Device in"=w5270) -> ("error out"=w5266:errorcluster, "State Machine.lvclass"=w5264:refnum<class "State Machine.lvclass">, "Device out"=w5269:refnum<class "Channel.lvclass">)  [unwired: 7 in]
            n2232 = call "Next State.vi"("error in (no error)"=w5266, "New_State"=12, "State Machine in"=w5264) -> ("error out"=w5265:errorcluster, "State Machine out"=w5263:refnum<class "State Machine.lvclass">)  [unwired: 7 in]
            n2233 = call-dynamic "Write State Machine.vi"("error in (no error)"=w5265, "State Machine.lvclass"=w5263, "Device in"=w5269) -> ("error out"=w5262:errorcluster, "Device out"=w5268:refnum<class "Channel.lvclass">)  [unwired: 7 in]
            n2234 = call-dynamic "Write Channel.vi"("error in (no error)"=w5262, "Channel.lvclass"=w5268, "Acquisition in"=w5286) -> ("error out"=w5284:errorcluster, "Acquisition out"=w5285:refnum<class "Acquisition.lvclass">)  [unwired: 7 in]
            n2235 = call-dynamic "Write AcquisitionA.vi"("error in (no error)"=w5284, "Acquisition.lvclass"=w5285, "S4ACS_GUI in"=w5287) -> ("error out"=w5282:errorcluster, "S4ACS_GUI out"=w5283:refnum<class "S4GUI.lvclass">)  [unwired: 7 in]
          }
          frame #1 {
            # "object"
            # "suffix"
            # "obsType"
            n2236 = call "Read AcquisitionB.vi"("error in (no error)"=w5340, "S4ACS_GUI in"=w5341) -> ("error out"=w5326:errorcluster, "Acquisition.lvclass"=w5327:refnum<class "Acquisition.lvclass">, "S4ACS_GUI out"=w5332:refnum<class "S4GUI.lvclass">)  [unwired: 7 in]
            n2237 = call-dynamic "Read Channel.vi"("error in (no error)"=w5326, "Acquisition in"=w5327) -> ("error out"=w5300:errorcluster, "Channel.lvclass"=w5302:refnum<class "Channel.lvclass">, "Acquisition out"=w5333:refnum<class "Acquisition.lvclass">)  [unwired: 7 in]
            n2238 = local read "Filter2"() -> (w5303:u8)
            n2239 = call-dynamic "Write Filter.vi"("error in (no error)"=w5300, "Filter"=w5303, "Channel in"=w5302) -> ("error out"=w5299:errorcluster, "Channel out"=w5301:refnum<class "Channel.lvclass">)  [unwired: 7 in]
            n2240 = call-dynamic "Read Interface.vi"("error in (no error)"=w5299, "Channel in"=w5301) -> ("error out"=w5314:errorcluster, "Interface.lvclass"=w5315:refnum<class "Interface.lvclass">, "Channel out"=w5328:refnum<class "Channel.lvclass">)  [unwired: 7 in]
            n2241 = call-dynamic "Write Suffix.vi"("error in (no error)"=w5314, "Suffix"=w5337, "Interface in"=w5315) -> ("error out"=w5323:errorcluster, "Interface out"=w5329:refnum<class "Interface.lvclass">)  [unwired: 7 in]
            n2242 = call-dynamic "Write ObsType.vi"("error in (no error)"=w5323, "ObsType"=w5322, "Interface in"=w5329) -> ("error out"=w5324:errorcluster, "Interface out"=w5330:refnum<class "Interface.lvclass">)  [unwired: 7 in]
            n2243 = call-dynamic "Write Object.vi"("error in (no error)"=w5324, "Object"=w5321, "Interface in"=w5330) -> ("error out"=w5325:errorcluster, "Interface out"=w5331:refnum<class "Interface.lvclass">)  [unwired: 7 in]
            n2244 = call-dynamic "Write Comments.vi"("error in (no error)"=w5325, "Comments"=w5336, "Interface in"=w5331) -> ("error out"=w5317:errorcluster, "Interface out"=w5316:refnum<class "Interface.lvclass">)  [unwired: 7 in]
            n2245 = call-dynamic "Write Observer.vi"("error in (no error)"=w5317, "Observer"=w5320, "Interface in"=w5316) -> ("error out"=w5318:errorcluster, "Interface out"=w5319:refnum<class "Interface.lvclass">)  [unwired: 7 in]
            n2246 = call-dynamic "Write Interface.vi"("error in (no error)"=w5318, "Interface.lvclass"=w5319, "Channel in"=w5328) -> ("error out"=w5307:errorcluster, "Channel out"=w5308:refnum<class "Channel.lvclass">)  [unwired: 7 in]
            n2247 = call-dynamic "Read State Machine.vi"("error in (no error)"=w5307, "Device in"=w5308) -> ("error out"=w5313:errorcluster, "State Machine.lvclass"=w5311:refnum<class "State Machine.lvclass">, "Device out"=w5306:refnum<class "Channel.lvclass">)  [unwired: 7 in]
            n2248 = call "Next State.vi"("error in (no error)"=w5313, "New_State"=12, "State Machine in"=w5311) -> ("error out"=w5312:errorcluster, "State Machine out"=w5310:refnum<class "State Machine.lvclass">)  [unwired: 7 in]
            n2249 = call-dynamic "Write State Machine.vi"("error in (no error)"=w5312, "State Machine.lvclass"=w5310, "Device in"=w5306) -> ("error out"=w5304:errorcluster, "Device out"=w5305:refnum<class "Channel.lvclass">)  [unwired: 7 in]
            n2250 = call-dynamic "Write Channel.vi"("error in (no error)"=w5304, "Channel.lvclass"=w5305, "Acquisition in"=w5333) -> ("error out"=w5335:errorcluster, "Acquisition out"=w5334:refnum<class "Acquisition.lvclass">)  [unwired: 7 in]
            n2251 = call "Write AcquisitionB.vi"("error in (no error)"=w5335, "Acquisition.lvclass"=w5334, "S4ACS_GUI in"=w5332) -> ("error out"=w5338:errorcluster, "S4ACS_GUI out"=w5339:refnum<class "S4GUI.lvclass">)  [unwired: 7 in]
          }
          frame #2 {
            # "object"
            # "suffix"
            # "obsType"
            n2252 = call-dynamic "Read AcquisitionC.vi"("error in (no error)"=w5383, "S4ACS_GUI in"=w5384) -> ("error out"=w5376:errorcluster, "Acquisition.lvclass"=w5375:refnum<class "Acquisition.lvclass">, "S4ACS_GUI out"=w5370:refnum<class "S4GUI.lvclass">)  [unwired: 7 in]
            n2253 = call-dynamic "Read Channel.vi"("error in (no error)"=w5376, "Acquisition in"=w5375) -> ("error out"=w5343:errorcluster, "Channel.lvclass"=w5345:refnum<class "Channel.lvclass">, "Acquisition out"=w5369:refnum<class "Acquisition.lvclass">)  [unwired: 7 in]
            n2254 = local read "Filter3"() -> (w5346:u8)
            n2255 = call-dynamic "Write Filter.vi"("error in (no error)"=w5343, "Filter"=w5346, "Channel in"=w5345) -> ("error out"=w5342:errorcluster, "Channel out"=w5344:refnum<class "Channel.lvclass">)  [unwired: 7 in]
            n2256 = call-dynamic "Read Interface.vi"("error in (no error)"=w5342, "Channel in"=w5344) -> ("error out"=w5361:errorcluster, "Interface.lvclass"=w5362:refnum<class "Interface.lvclass">, "Channel out"=w5374:refnum<class "Channel.lvclass">)  [unwired: 7 in]
            n2257 = call-dynamic "Write Suffix.vi"("error in (no error)"=w5361, "Suffix"=w5380, "Interface in"=w5362) -> ("error out"=w5379:errorcluster, "Interface out"=w5373:refnum<class "Interface.lvclass">)  [unwired: 7 in]
